vi "Self Configure.vi"(8 "error in":errorcluster, 11 "Electronic Load in":refnum<class "Electronic Load.lvclass">) -> (0 "error out":errorcluster, 3 "Electronic Load out":refnum<class "Electronic Load.lvclass">)   [LabVIEW 2019, in "Electronic Load.lvlib" / "Electronic Load.lvclass"]
uses:
  Library/Electronic Load.lvclass
  Custom Controls/Configuration Keys.ctl
  Library/Electronic Load.lvclass/Electronic Load.ctl
  Accessors/Write Available Channels.vi
  builds/Instruments/Instruments.lvlibp/Library/Instruments.lvclass
  builds/Tools/Config.lvlibp/Config.lvclass
  C:/Users/Public/Documents/Development/builds/Tools/Config.lvlibp/Config.lvclass
panel:
  in  "Configuration Keys":T1
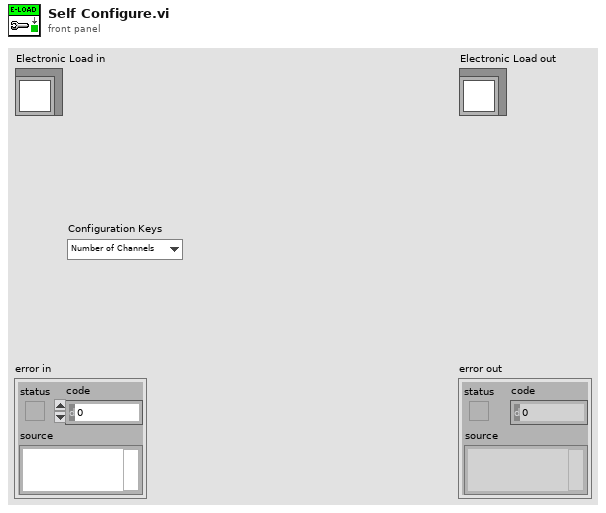
[diagram p1: front panel]
types:
  T1 = typedef "Electronic Load.lvlib/Electronic Load.lvclass/Configuration Keys.ctl" = enum16{"Number of Channels"}
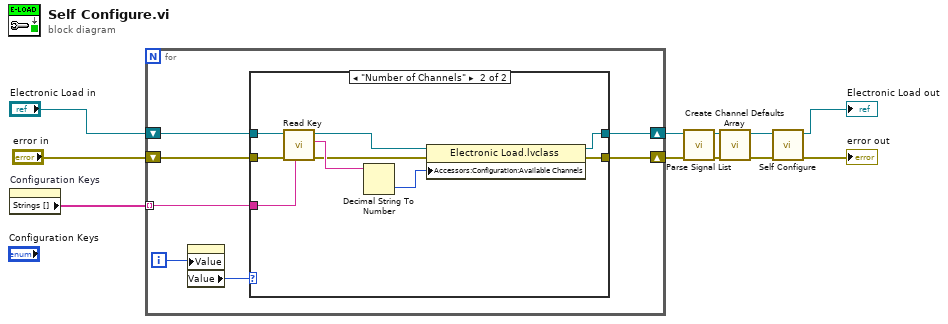
[diagram p0: block diagram]
diagram:
  n1 = property on="Configuration Keys" class="Enum (strict)"() -> ("Strings []"=w11:string[])  [unwired: 2 in, 2 out]
  n2 = for {
    tunnel: w11 -> [w16] mode=indexing
    shift-right: [w14] -> w4
    shift-left: "Electronic Load in" -> [w15]
    shift-right: [w12] -> w3
    shift-left: "error in" -> [w13]
    i -> [w18]
    n3 = property on="Configuration Keys" class="Enum (strict)"("Value"=w18) -> ("Value"=w17:T1)  [unwired: 2 in, 2 out]
    n4 = case shown="\"Number of Channels\"" w17 {
      tunnel: w16 -> [_ w22]
      tunnel: w15 -> [w20 w25]
      tunnel: [w20 w21] -> w14
      tunnel: w13 -> [w19 w24]
      tunnel: [w19 w23] -> w12
      frame Default {
      }
      frame "Number of Channels" {
        n5 = call "Read Key.vi"("Key Name"=w22, "error in"=w24, "Config in"=w25) -> ("error out"=w28:errorcluster, "Key Value"=w29:string, "Config out"=w27:refnum<class "Electronic Load.lvclass">)  [unwired: 6 in]
        n6 = Decimal String To Number(string=w29) -> (number=w26:i32)  [unwired: 2 in, 1 out]
        n7 = property class="Electronic Load.lvclass"(reference=w27, error in=w28, "Accessors:Configuration:Available Channels"=w26) -> (reference out=w21:refnum<class "Electronic Load.lvclass">, error out=w23:errorcluster)
      }
    }
  }
  n8 = call "Parse Signal List.vi"("error in"=w3, "Electronic Load in"=w4) -> ("error out"=w1:errorcluster, "Electronic Load out"=w2:refnum<class "Electronic Load.lvclass">)  [unwired: 8 in]
  n9 = call "Create Channel Defaults Array.vi"("error in"=w1, "Electronic Load in"=w2) -> ("error out"=w7:errorcluster, "Electronic Load out"=w8:refnum<class "Electronic Load.lvclass">)  [unwired: 8 in]
  n10 = call-parent "Self Configure.vi"("error in"=w7, "Instruments in"=w8) -> ("error out"=→"error out":errorcluster, "Instruments out"=→"Electronic Load out":refnum<class "Electronic Load.lvclass">)  [unwired: 8 in]
